vi "Read Waveform Type.vi"(8 "error in (no error)":errorcluster, 11 "Advanced Waveform in":refnum<class "Advanced Waveform.lvclass">) -> (0 "error out":errorcluster, 2 "Waveform Type":T1, 3 "Advanced Waveform out":refnum<class "Advanced Waveform.lvclass">)   [LabVIEW 2011, in "Advanced Waveform.lvclass"]
uses:
  Advanced Waveform.lvclass
  Controls/Waveform Type.ctl
  Advanced Waveform.lvclass/Advanced Waveform.ctl
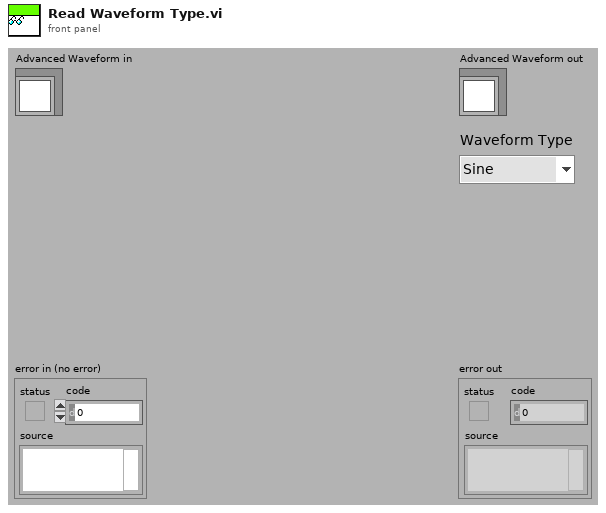
[diagram p1: front panel]
types:
  T1 = typedef "Waveform Type.ctl" = enum16{"Sine", "Square", "Triangle"}
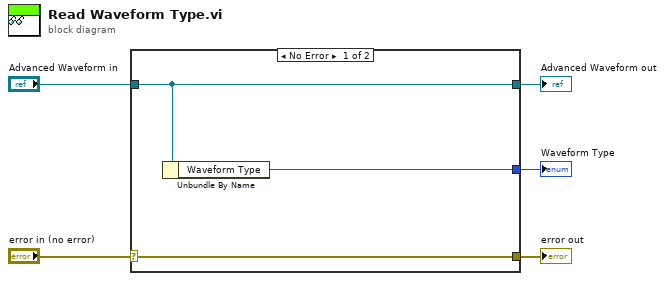
[diagram p0: block diagram]
diagram:
  n1 = case shown="No Error" "error in (no error)" {
    selector: "error in (no error)" -> [w8 w9]
    tunnel: [w8 w9] -> w4
    tunnel: [w7 w10] -> w2
    tunnel: "Advanced Waveform in" -> [w7 w10]
    tunnel: [w6 _] -> w1
    frame No Error {
      n2 = Unbundle By Name(w7) -> ("Waveform Type"=w6:T1)
    }
    frame Error {
    }
  }
  "error out" <- w4
  "Advanced Waveform out" <- w2
  "Waveform Type" <- w1
